vi "报表生成_word书签插入.vi"() -> ()   [LabVIEW 2020]
uses:
  <vilib>/Utility/NIReport.llb/Report Type.ctl
  <vilib>/Utility/NIReport.llb/Append Report Text (str wrap).vi
  <vilib>/Utility/NIReport.llb/Append Text Table to Report (wrap).vi
  <vilib>/Utility/NIReport.llb/NI_report.lvclass
  <vilib>/Utility/NIReport.llb/NI_ReportGenerationCore.lvlib
panel:
  in  "report file path":path caption="报表文件路径"
  out "error out":errorcluster caption="错误输出"
  in  "template (empty)":path caption="模板（空）"
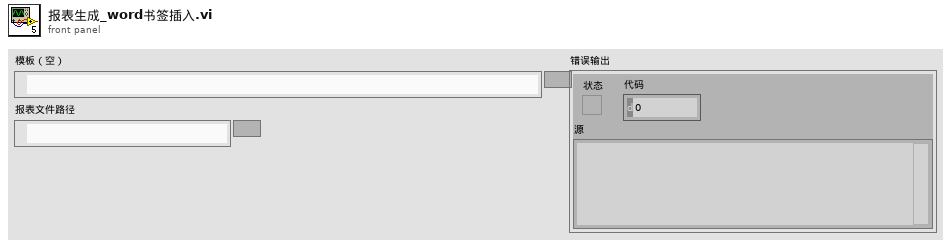
[diagram p1: front panel]
types:
  T1 = cluster{"position (excel)":cluster{"row":i32, "column":i32}, "name (excel)":string, "bookmark (word)":string}
  T2 = typedef "NI_ReportGenerationCore.lvlib/Report Type.ctl" = enum16{"HTML", "Word", "Excel"}
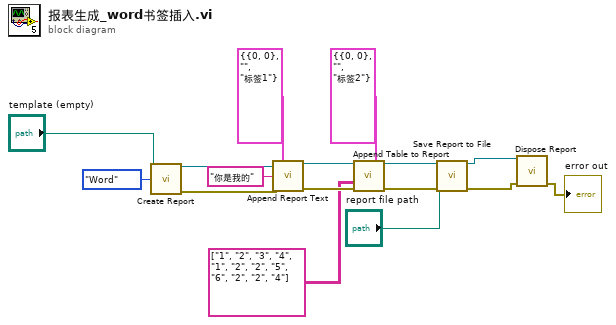
[diagram p0: block diagram]
diagram:
  n1 = call <vilib>:"Create Report.vi"("report type"=Report_Type."Word", "template (empty)"="template (empty)") -> ("report out"=w14:refnum<class "NI_report.lvclass">, "error out"=w13:errorcluster)  [unwired: 12 in]
  n2 = call-poly <vilib>:"Append Report Text.vi"("report in"=w14, "MS Office parameters"=T1 {"position (excel)"={"row"=0, "column"=0}, "name (excel)"="", "bookmark (word)"="标签1"}, "text"="你是我的", "error in (no error)"=w13) -> ("report out"=w10:refnum<class "NI_report.lvclass">, "error out"=w9:errorcluster)  [unwired: 8 in, 2 out]
  n3 = call-poly <vilib>:"Append Table to Report.vi"("report in"=w10, "MS Office parameters"=T1 {"position (excel)"={"row"=0, "column"=0}, "name (excel)"="", "bookmark (word)"="标签2"}, "text data"=string[][] [["1", "2", "3", "4"], ["1", "2", "2", "5"], ["6", "2", "2", "4"]], "error in (no error)"=w9) -> ("report out"=w7:refnum<class "NI_report.lvclass">, "error out"=w8:errorcluster)  [unwired: 8 in, 2 out]
  n4 = call-dynamic "Save Report to File.vi"("report in"=w7, "report file path"="report file path", "error in (no error)"=w8) -> ("report out"=w4:refnum<class "NI_report.lvclass">, "error out"=w3:errorcluster)  [unwired: 11 in]
  n5 = call-dynamic "Dispose Report.vi"("report in"=w4, "error in (no error)"=w3) -> ("error out"=→"error out":errorcluster)  [unwired: 13 in]
